vi "random walk (behavior).vi"(4 "possible drive vectors":i8[](array[numeric])=[0, 0, 0, 0, 0, 0, 0, 0, 0]) -> (1 "selected drive vector":i8)   [LabVIEW 2009]
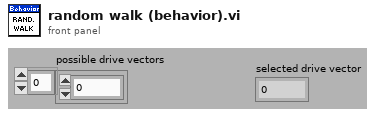
[diagram p1: front panel]
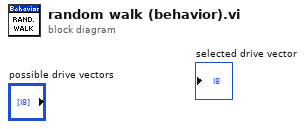
[diagram p0: block diagram]
diagram:
